vi "TEST_ContextMenuRTM.vi"() -> ()   [LabVIEW 2021]
uses:
  Menu.lvclass
  MenuSelection.ctl
  Picture2D/src/Color/Color.lvclass
  SubMenuIcon.ctl
  Picture2D/src/Circle/Circle.lvclass
  C:/GitHub/Picture2D/src/Picture2D/Picture2D.lvclass
  C:/GitHub/Picture2D/src/Shape/Shape.lvclass
  Picture2D/src/Point/Point.lvclass
  975e9a7f-0e71-4990-a718-d11c6985bb5a.vi
  Picture2D/src/Picture/Image.lvclass
  SetBackgroundColor.vi
  SetBorderColor.vi
  SetHiliteColor.vi
  SetHiliteTextColor.vi
  SetTextColor.vi
  SetSubMenuIconType.vi
  SetSubMenuIconOpened.vi
  SetSubMenuIconClosed.vi
  <vilib>/ErrorRing/Error Ring.xnode
panel:
  in  "SubMenuIconType":enum16{"LabVIEW", "Windows", "Custom"}(ring)
  in  "Right click me":string
  in  "Color Theme":enum16{"LabVIEW", "Dark", "Windows Gray"}(ring)
  out "ItemPath":string
  out "ItemTag":string
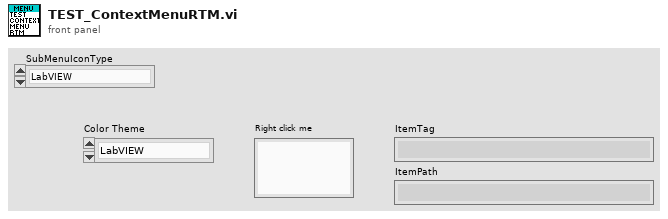
[diagram p1: front panel]
types:
  T1 = typedef "Menu.lvlib/Menu.lvclass/SubMenuIcon.ctl" = enum16{"LabVIEW", "Windows", "Custom"}
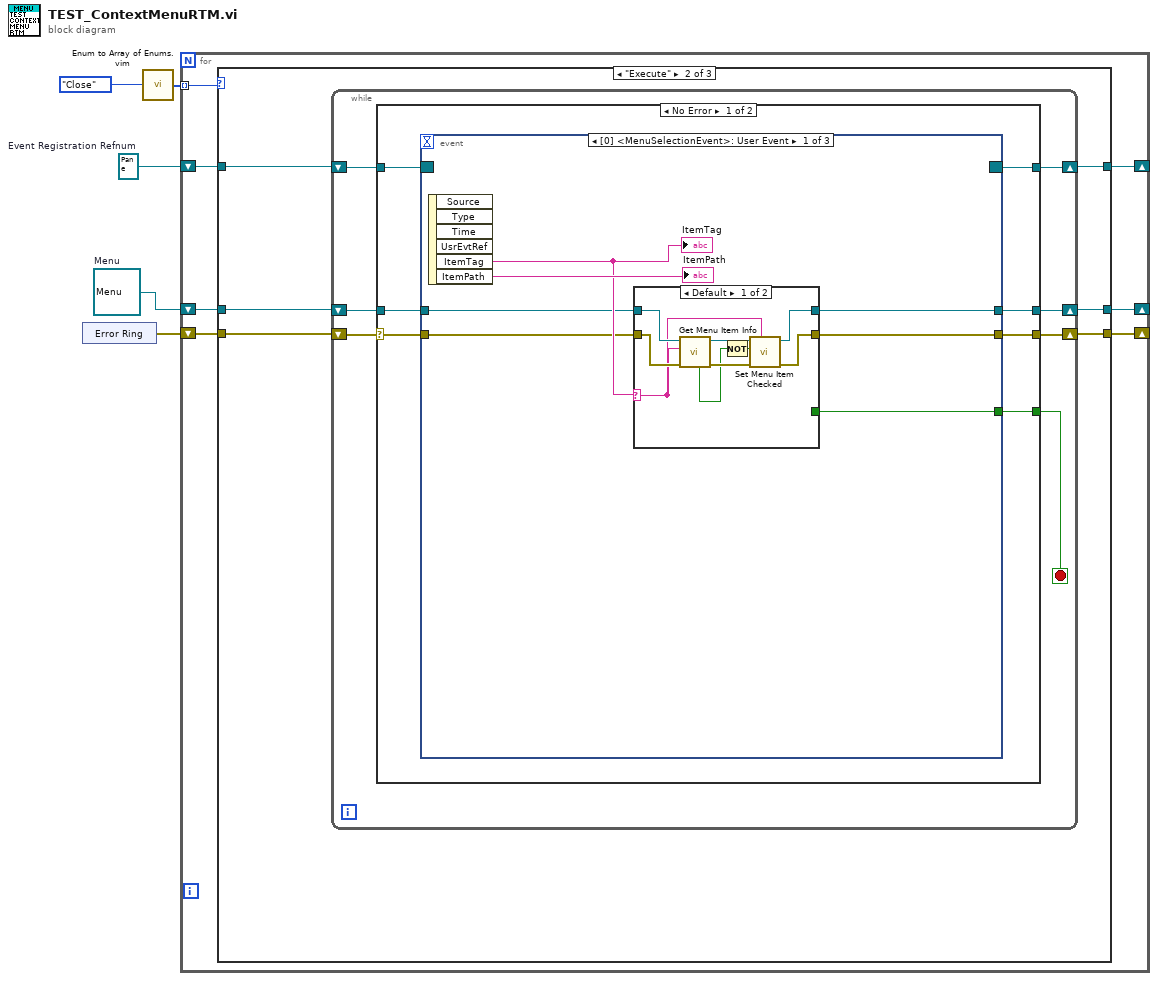
[diagram p0: block diagram]
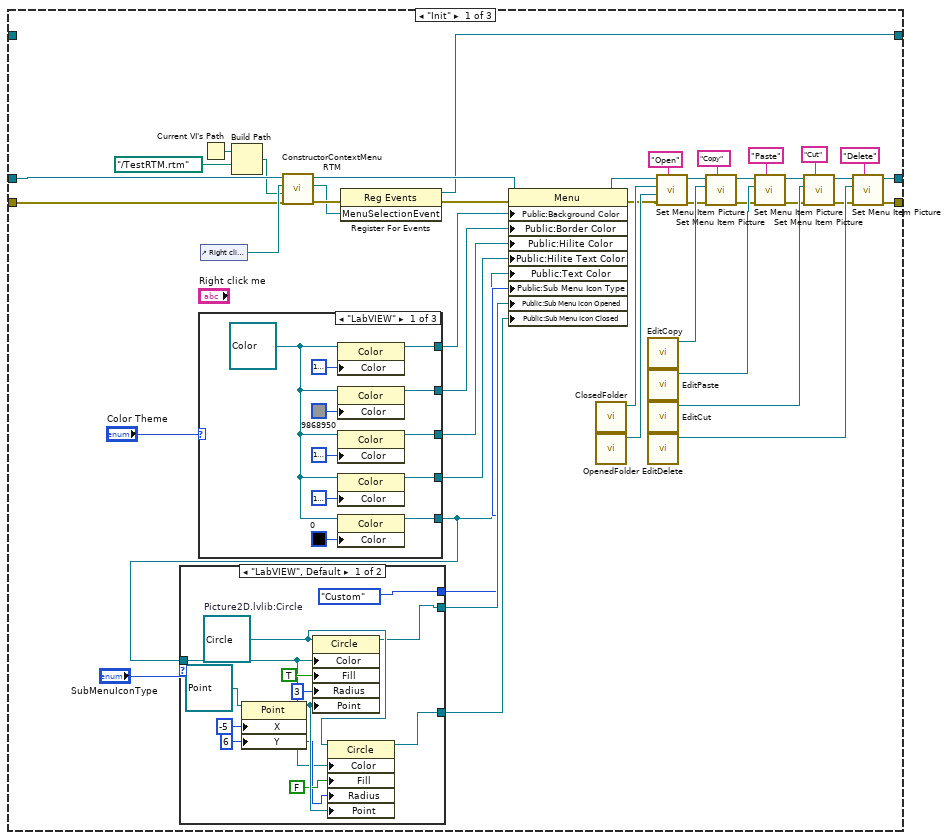
[diagram p2: hidden frame]
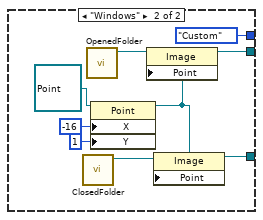
[diagram p3: hidden frame]
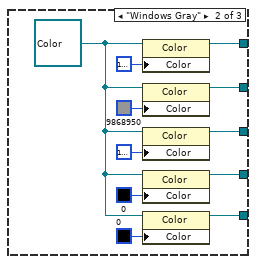
[diagram p4: hidden frame]
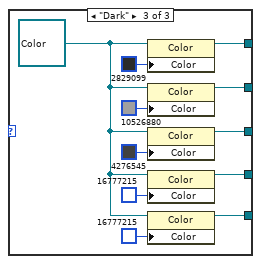
[diagram p5: hidden frame]
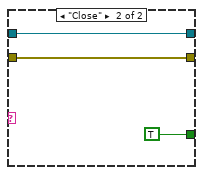
[diagram p6: hidden frame]
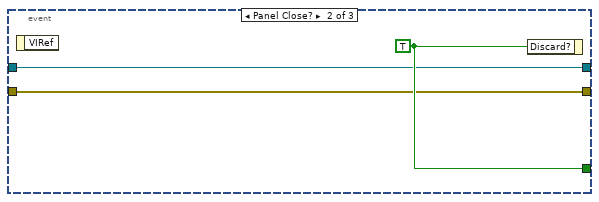
[diagram p7: hidden frame]
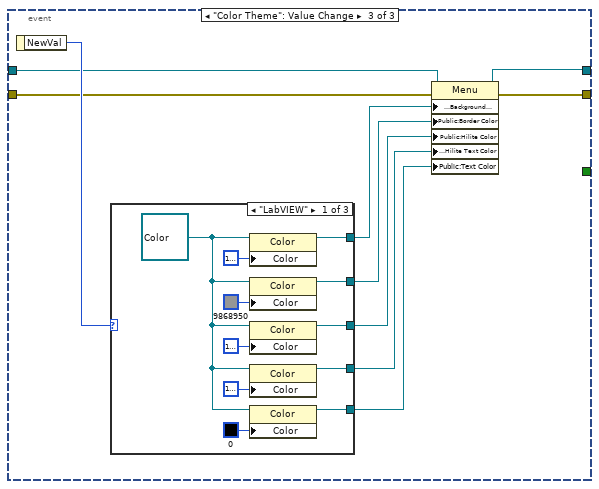
[diagram p8: hidden frame]
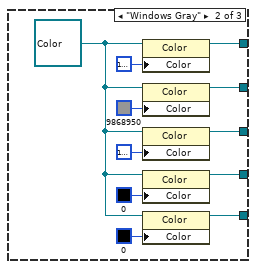
[diagram p9: hidden frame]
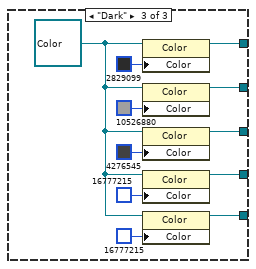
[diagram p10: hidden frame]
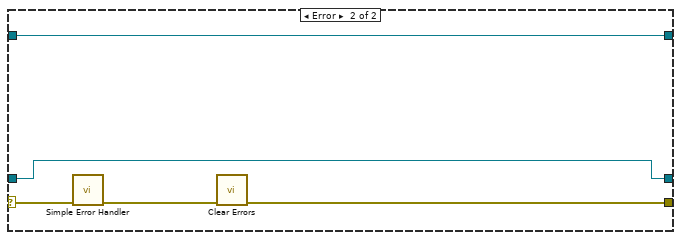
[diagram p11: hidden frame]
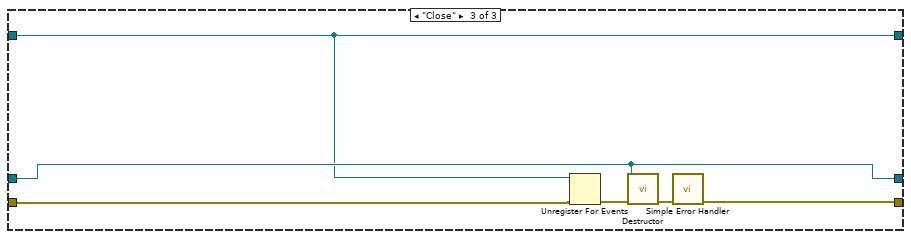
[diagram p12: hidden frame]
diagram:
  w5 = refnum<event-registration> refnum  # Event Registration Refnum
  w2 = refnum<class "Menu.lvclass"> refnum  # Menu
  n1 = xnode "Error Ring"() -> ("error out"=w1:errorcluster)
  n2 = call "Enum to Array of Enums.vim"("enum"=enum16{"Init", "Execute", "Close"}."Close") -> ("array of enums"=w3:enum16{"Init", "Execute", "Close"}[])
  n3 = for {
    shift-right: [w6] -> _
    shift-left: w5 -> [w12]
    shift-right: [w8] -> _
    shift-left: w1 -> [w11]
    shift-right: [w7] -> _
    shift-left: w2 -> [w10]
    tunnel: w3 -> [w9] mode=indexing
    n4 = case shown="\"Execute\"" w9 {
      tunnel: w12 -> [_ w116 w201]
      tunnel: [w38 w115 w202] -> w7
      tunnel: [w23 w114 w201] -> w6
      tunnel: [w37 w113 w203] -> w8
      tunnel: w11 -> [w25 w112 w204]
      tunnel: w10 -> [w24 w111 w202]
      frame "Init" {
        n5 = case shown="\"LabVIEW\"" "Color Theme" {
          tunnel: [w88 w99 w110] -> w30
          tunnel: [w86 w97 w108] -> w31
          tunnel: [w85 w96 w107] -> w32
          tunnel: [w84 w95 w106] -> w33
          tunnel: [w83 w94 w100] -> w13
          frame "LabVIEW" {
            w87 = refnum<class "Color.lvclass"> refnum ("Background Color")
            n6 = property class="Color"(reference=w87, "Color"=u32 16777238) -> (reference out=w88:refnum<class "Color.lvclass">)  [unwired: 1 in, 1 out]
            n7 = property class="Color"(reference=w87, "Color"=u32 9868950) -> (reference out=w86:refnum<class "Color.lvclass">)  [unwired: 1 in, 1 out]
            n8 = property class="Color"(reference=w87, "Color"=u32 16777224) -> (reference out=w85:refnum<class "Color.lvclass">)  [unwired: 1 in, 1 out]
            n9 = property class="Color"(reference=w87, "Color"=u32 16777226) -> (reference out=w84:refnum<class "Color.lvclass">)  [unwired: 1 in, 1 out]
            n10 = property class="Color"(reference=w87, "Color"=u32 0) -> (reference out=w83:refnum<class "Color.lvclass">)  [unwired: 1 in, 1 out]
          }
          frame "Windows Gray" {
            w98 = refnum<class "Color.lvclass"> refnum ("Background Color")
            n11 = property class="Color"(reference=w98, "Color"=u32 16777238) -> (reference out=w99:refnum<class "Color.lvclass">)  [unwired: 1 in, 1 out]
            n12 = property class="Color"(reference=w98, "Color"=u32 9868950) -> (reference out=w97:refnum<class "Color.lvclass">)  [unwired: 1 in, 1 out]
            n13 = property class="Color"(reference=w98, "Color"=u32 16777225) -> (reference out=w96:refnum<class "Color.lvclass">)  [unwired: 1 in, 1 out]
            n14 = property class="Color"(reference=w98, "Color"=u32 0) -> (reference out=w95:refnum<class "Color.lvclass">)  [unwired: 1 in, 1 out]
            n15 = property class="Color"(reference=w98, "Color"=u32 0) -> (reference out=w94:refnum<class "Color.lvclass">)  [unwired: 1 in, 1 out]
          }
          frame "Dark" {
            w109 = refnum<class "Color.lvclass"> refnum ("Background Color")
            n16 = property class="Color"(reference=w109, "Color"=u32 2829099) -> (reference out=w110:refnum<class "Color.lvclass">)  [unwired: 1 in, 1 out]
            n17 = property class="Color"(reference=w109, "Color"=u32 10526880) -> (reference out=w108:refnum<class "Color.lvclass">)  [unwired: 1 in, 1 out]
            n18 = property class="Color"(reference=w109, "Color"=u32 4276545) -> (reference out=w107:refnum<class "Color.lvclass">)  [unwired: 1 in, 1 out]
            n19 = property class="Color"(reference=w109, "Color"=u32 16777215) -> (reference out=w106:refnum<class "Color.lvclass">)  [unwired: 1 in, 1 out]
            n20 = property class="Color"(reference=w109, "Color"=u32 16777215) -> (reference out=w100:refnum<class "Color.lvclass">)  [unwired: 1 in, 1 out]
          }
        }
        n21 = case shown="\"LabVIEW\", Default" "SubMenuIconType" {
          tunnel: [w59 w71] -> w16
          tunnel: [w60 w70] -> w15
          tunnel: [SubMenuIcon."Custom" ("SubMenuIconType") SubMenuIcon."Custom" ("SubMenuIconType")] -> w14
          tunnel: w13 -> [w57 _]
          frame "LabVIEW", Default {
            w65 = i16 3 ("Radius")
            w67 = refnum<class "Circle.lvclass"> refnum  # Picture2D.lvlib:Circle
            n22 = property class="Point"(reference=refnum<class "Point.lvclass"> refnum ("Point"), "X"=i16 -5, "Y"=i16 6) -> (reference out=w68:refnum<class "Point.lvclass">)  [unwired: 1 in, 1 out]
            n23 = property class="Circle"(reference=w67, "Color"=w57, "Fill"=TRUE, "Radius"=w65, "Point"=w68) -> (reference out=w60:refnum<class "Circle.lvclass">)  [unwired: 1 in, 1 out]
            n24 = property class="Circle"(reference=w67, "Color"=w57, "Fill"=FALSE, "Radius"=w65, "Point"=w68) -> (reference out=w59:refnum<class "Circle.lvclass">)  [unwired: 1 in, 1 out]
          }
          frame "Windows" {
            n25 = call "ClosedFolder.vi"() -> ("Image out"=w76:refnum<class "Image.lvclass">)  [unwired: 11 in]
            n26 = call "OpenedFolder.vi"() -> ("Image out"=w77:refnum<class "Image.lvclass">)  [unwired: 11 in]
            n27 = property class="Point"(reference=refnum<class "Point.lvclass"> refnum ("Point"), "X"=i16 -16, "Y"=i16 1) -> (reference out=w75:refnum<class "Point.lvclass">)  [unwired: 1 in, 1 out]
            n28 = property class="Image"(reference=w77, "Point"=w75) -> (reference out=w70:refnum<class "Image.lvclass">)  [unwired: 1 in, 1 out]
            n29 = property class="Image"(reference=w76, "Point"=w75) -> (reference out=w71:refnum<class "Image.lvclass">)  [unwired: 1 in, 1 out]
          }
        }
        n30 = Current VI's Path() -> (path=w20:path)
        n31 = control-ref of="Right click me"() -> (w35:refnum<vi>)
        n32 = Build Path(base path=w20, name or relative path=path "../TestRTM.rtm" ("Path")) -> (appended path=w18:path)
        n33 = call "ConstructorContextMenuRTM.vi"("error in (no error)"=w25, "RTM Path"=w18, "CtrlRef"=w35, "Menu in"=w24) -> ("error out"=w28:errorcluster, "MenuSelectionEvent"=w26:refnum<user-event>, "Menu out"=w29:refnum<class "Menu.lvclass">)  [unwired: 5 in]
        n34 = register-events(error in=w28, w26) -> (reference out=w23:refnum<event-registration>, error out=w27:errorcluster)  [unwired: 1 in]
        n35 = property class="Menu"(reference=w29, error in=w27, "Public:Background Color"=w30, "Public:Border Color"=w31, "Public:Hilite Color"=w32, "Public:Hilite Text Color"=w33, "Public:Text Color"=w13, "Public:Sub Menu Icon Type"=w14, "Public:Sub Menu Icon Opened"=w15, "Public:Sub Menu Icon Closed"=w16) -> (reference out=w21:refnum<class "Menu.lvclass">, error out=w22:errorcluster)
        n36 = call "ClosedFolder.vi"() -> ("Image out"=w55:refnum<class "Image.lvclass">)  [unwired: 11 in]
        n37 = call "OpenedFolder.vi"() -> ("Image out"=w56:refnum<class "Image.lvclass">)  [unwired: 11 in]
        n38 = call "EditCopy.vi"() -> ("Image out"=w51:refnum<class "Image.lvclass">)  [unwired: 11 in]
        n39 = call "EditPaste.vi"() -> ("Image out"=w52:refnum<class "Image.lvclass">)  [unwired: 11 in]
        n40 = call "EditCut.vi"() -> ("Image out"=w53:refnum<class "Image.lvclass">)  [unwired: 11 in]
        n41 = call "EditDelete.vi"() -> ("Image out"=w54:refnum<class "Image.lvclass">)  [unwired: 11 in]
        n42 = call "Set Menu Item Picture.vi"("item tag"="Open", "error in (no error)"=w22, "Hilite Picture"=w56, "Picture"=w55, "Menu in"=w21) -> ("error out"=w41:errorcluster, "Menu out"=w40:refnum<class "Menu.lvclass">)  [unwired: 5 in]
        n43 = call "Set Menu Item Picture.vi"("item tag"="Copy", "error in (no error)"=w41, "Picture"=w51, "Menu in"=w40) -> ("error out"=w43:errorcluster, "Menu out"=w42:refnum<class "Menu.lvclass">)  [unwired: 6 in]
        n44 = call "Set Menu Item Picture.vi"("item tag"="Paste", "error in (no error)"=w43, "Picture"=w52, "Menu in"=w42) -> ("error out"=w45:errorcluster, "Menu out"=w44:refnum<class "Menu.lvclass">)  [unwired: 6 in]
        n45 = call "Set Menu Item Picture.vi"("item tag"="Cut", "error in (no error)"=w45, "Picture"=w53, "Menu in"=w44) -> ("error out"=w47:errorcluster, "Menu out"=w46:refnum<class "Menu.lvclass">)  [unwired: 6 in]
        n46 = call "Set Menu Item Picture.vi"("item tag"="Delete", "error in (no error)"=w47, "Picture"=w54, "Menu in"=w46) -> ("error out"=w37:errorcluster, "Menu out"=w38:refnum<class "Menu.lvclass">)  [unwired: 6 in]
      }
      frame "Execute" {
        n47 = while {
          shift-right: [w121] -> w113
          shift-left: w112 -> [w122]
          shift-right: [w118] -> w114
          shift-left: w116 -> [w123]
          shift-right: [w119] -> w115
          shift-left: w111 -> [w120]
          stop <- w117 stop-if-true
          n48 = case shown="No Error" w122 {
            selector: w122 -> [w129 w200]
            tunnel: w123 -> [w130 w199]
            tunnel: [w128 w196] -> w121
            tunnel: w120 -> [w127 w198]
            tunnel: [w126 w198] -> w119
            tunnel: [w125 w199] -> w118
            tunnel: [w124 _] -> w117
            frame No Error {
              n49 = event shown="[0] <MenuSelectionEvent>: User Event" {
                selector: w130 -> [_ _ _]
                dyn-events: [_ _ _] -> w125
                timeout: _ -> [_ _ _]
                tunnel: [w132 w151 w155] -> w128
                tunnel: w129 -> [w133 w151 w156]
                tunnel: [w131 w150 w153] -> w126
                tunnel: w127 -> [w134 w150 w154]
                tunnel: [w135 w152 _] -> w124
                event User Event {
                  n50 = event-data() -> ("ItemTag"=w136:string, "ItemPath"=→"ItemPath":string)  [unwired: 1 in, 4 out]
                  "ItemTag" <- w136
                  n51 = case shown="Default" w136 {
                    selector: w136 -> [w138 _]
                    tunnel: [_ TRUE] -> w135
                    tunnel: w134 -> [w146 w148]
                    tunnel: w133 -> [w145 w147]
                    tunnel: [w143 w147] -> w132
                    tunnel: [w141 w148] -> w131
                    frame Default {
                      n52 = call "Get Menu Item Info.vi"("error in (no error)"=w145, "item tag"=w138, "Menu in"=w146) -> ("error out"=w144:errorcluster, "Menu out"=w142:refnum<class "Menu.lvclass">, "checked"=w140:bool)  [unwired: 1 in, 5 out]
                      n53 = Not(x=w140) -> (.not. x?=w139:bool)
                      n54 = call "Set Menu Item Checked.vi"("item tag"=w138, "error in (no error)"=w144, "checked"=w139, "Menu in"=w142) -> ("error out"=w143:errorcluster, "Menu out"=w141:refnum<class "Menu.lvclass">)  [unwired: 6 in]
                    }
                    frame "Close" {
                    }
                  }
                }
                event Panel Close? {
                  w152 = TRUE ("Discard?")
                  n55 = event-data() -> ()  [unwired: 1 in, 1 out]
                  n56 = event-data("Discard?"=w152) -> ()  [unwired: 1 in, 1 out]
                }
                event "Color Theme": Value Change {
                  n57 = event-data() -> ("NewVal"=w157:enum16{"LabVIEW", "Dark", "Windows Gray"})  [unwired: 1 in]
                  n58 = case shown="\"LabVIEW\"" w157 {
                    tunnel: [w173 w184 w195] -> w162
                    tunnel: [w171 w182 w193] -> w161
                    tunnel: [w170 w181 w192] -> w160
                    tunnel: [w169 w180 w191] -> w159
                    tunnel: [w168 w179 w190] -> w158
                    frame "LabVIEW" {
                      w172 = refnum<class "Color.lvclass"> refnum ("Background Color")
                      n59 = property class="Color"(reference=w172, "Color"=u32 16777238) -> (reference out=w173:refnum<class "Color.lvclass">)  [unwired: 1 in, 1 out]
                      n60 = property class="Color"(reference=w172, "Color"=u32 9868950) -> (reference out=w171:refnum<class "Color.lvclass">)  [unwired: 1 in, 1 out]
                      n61 = property class="Color"(reference=w172, "Color"=u32 16777224) -> (reference out=w170:refnum<class "Color.lvclass">)  [unwired: 1 in, 1 out]
                      n62 = property class="Color"(reference=w172, "Color"=u32 16777226) -> (reference out=w169:refnum<class "Color.lvclass">)  [unwired: 1 in, 1 out]
                      n63 = property class="Color"(reference=w172, "Color"=u32 0) -> (reference out=w168:refnum<class "Color.lvclass">)  [unwired: 1 in, 1 out]
                    }
                    frame "Windows Gray" {
                      w183 = refnum<class "Color.lvclass"> refnum ("Background Color")
                      n64 = property class="Color"(reference=w183, "Color"=u32 16777238) -> (reference out=w184:refnum<class "Color.lvclass">)  [unwired: 1 in, 1 out]
                      n65 = property class="Color"(reference=w183, "Color"=u32 9868950) -> (reference out=w182:refnum<class "Color.lvclass">)  [unwired: 1 in, 1 out]
                      n66 = property class="Color"(reference=w183, "Color"=u32 16777225) -> (reference out=w181:refnum<class "Color.lvclass">)  [unwired: 1 in, 1 out]
                      n67 = property class="Color"(reference=w183, "Color"=u32 0) -> (reference out=w180:refnum<class "Color.lvclass">)  [unwired: 1 in, 1 out]
                      n68 = property class="Color"(reference=w183, "Color"=u32 0) -> (reference out=w179:refnum<class "Color.lvclass">)  [unwired: 1 in, 1 out]
                    }
                    frame "Dark" {
                      w194 = refnum<class "Color.lvclass"> refnum ("Background Color")
                      n69 = property class="Color"(reference=w194, "Color"=u32 2829099) -> (reference out=w195:refnum<class "Color.lvclass">)  [unwired: 1 in, 1 out]
                      n70 = property class="Color"(reference=w194, "Color"=u32 10526880) -> (reference out=w193:refnum<class "Color.lvclass">)  [unwired: 1 in, 1 out]
                      n71 = property class="Color"(reference=w194, "Color"=u32 4276545) -> (reference out=w192:refnum<class "Color.lvclass">)  [unwired: 1 in, 1 out]
                      n72 = property class="Color"(reference=w194, "Color"=u32 16777215) -> (reference out=w191:refnum<class "Color.lvclass">)  [unwired: 1 in, 1 out]
                      n73 = property class="Color"(reference=w194, "Color"=u32 16777215) -> (reference out=w190:refnum<class "Color.lvclass">)  [unwired: 1 in, 1 out]
                    }
                  }
                  n74 = property class="Menu"(reference=w154, error in=w156, "Public:Background Color"=w162, "Public:Border Color"=w161, "Public:Hilite Color"=w160, "Public:Hilite Text Color"=w159, "Public:Text Color"=w158) -> (reference out=w153:refnum<class "Menu.lvclass">, error out=w155:errorcluster)
                }
              }
            }
            frame Error {
              n75 = call <vilib>:"Simple Error Handler.vi"("error in (no error)"=w200) -> ("error out"=w197:errorcluster)  [unwired: 4 in, 4 out]
              n76 = call <vilib>:"Clear Errors.vi"("error in (no error)"=w197) -> ("error out"=w196:errorcluster)  [unwired: 5 in, 1 out]
            }
          }
        }
      }
      frame "Close" {
        n77 = Unregister For Events(event registration refnum=w201, error in=w204) -> (error out=w205:errorcluster)
        n78 = call "Destructor.vi"("error in (no error)"=w205, "Menu in"=w202) -> ("error out"=w206:errorcluster)  [unwired: 9 in]
        n79 = call <vilib>:"Simple Error Handler.vi"("error in (no error)"=w206) -> ("error out"=w203:errorcluster)  [unwired: 4 in, 4 out]
      }
    }
  }
